vi "ScanAction.vi"(8 "error in (no error)":errorcluster caption="entrée d'erreur (pas d'erreur)", 9 "IndicePoint":i32, 10 "Dir":bool, 11 "Tools In":refnum<class "CoboltMLD.lvclass"> caption="DNL_LabVIEW Object in") -> (0 "error out":errorcluster caption="sortie d'erreur", 2 "ScanParsOut":dbl[](array[numeric]), 3 "Tools Out":refnum<class "CoboltMLD.lvclass"> caption="DNL_LabVIEW Object out")   [LabVIEW 2019, in "CoboltMLD.lvclass"]
uses:
  CoboltMLD.lvclass
  C:/Programmes Labview/LabscanV1A/DevicesClass/BaseDevice/BaseDevice.lvclass
  CoboltMLD.lvclass/CoboltMLD.ctl
  <userlib>/GenProg/ReadValByRefU32.vi
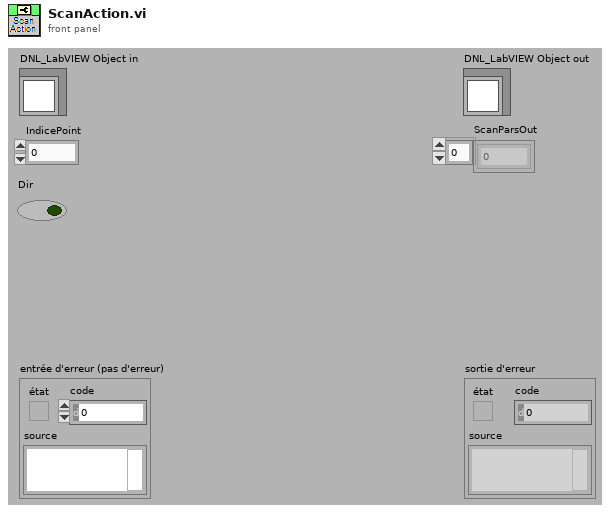
[diagram p1: front panel]
types:
  T1 = typedef "CoboltMLD.lvclass/CoboltMLD_Func.ctl" = enum16{"Power (mW)", "Freq (kHz)"}
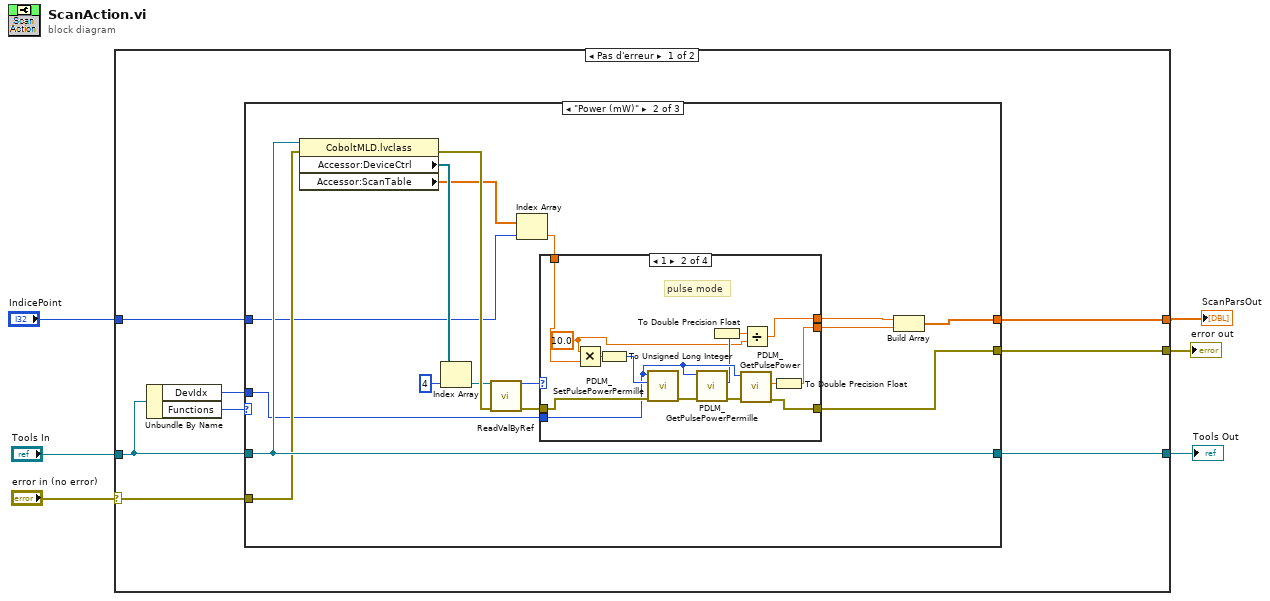
[diagram p0: block diagram]
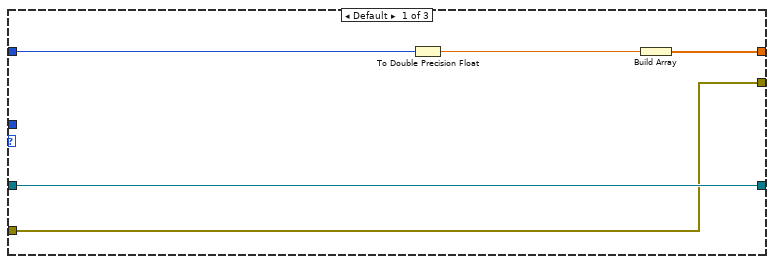
[diagram p2: hidden frame]
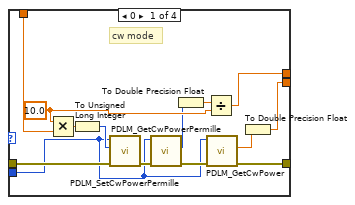
[diagram p3: hidden frame]
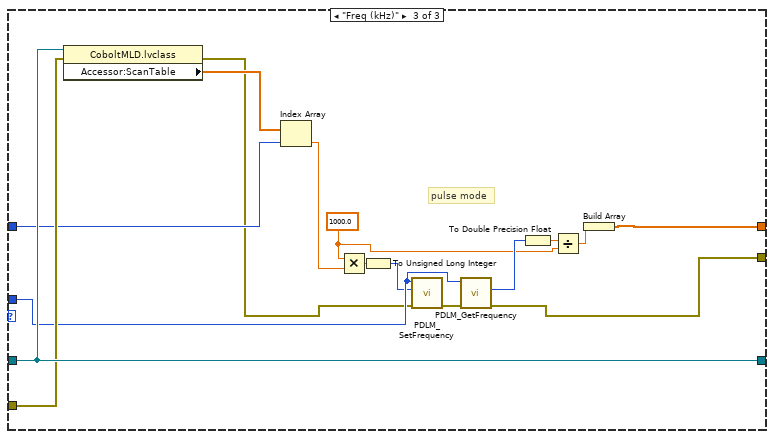
[diagram p6: hidden frame]
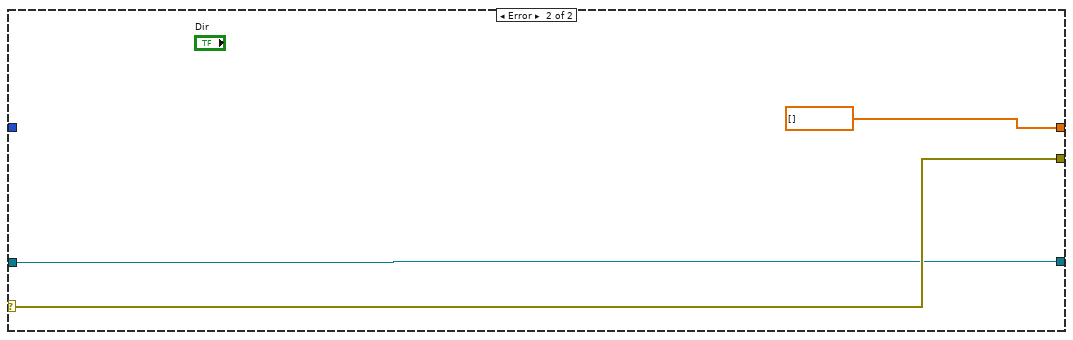
[diagram p7: hidden frame]
diagram:
  n1 = case shown="Pas d'erreur" "error in (no error)" {
    selector: "error in (no error)" -> [w11 w84]
    tunnel: "Tools In" -> [w12 w83]
    tunnel: [w10 dbl[] []] -> w1
    tunnel: [w9 w84] -> w4
    tunnel: [w8 w83] -> w3
    tunnel: "IndicePoint" -> [w13 _]
    frame No Error {
      n2 = Unbundle By Name(w12) -> ("DevIdx"=w7:i32, "Functions"=w14:T1)
      n3 = case shown="\"Power (mW)\"" w14 {
        tunnel: [w15 w35 w74] -> w10
        tunnel: w13 -> [w19 w26 w78]
        tunnel: [w17 w34 w81] -> w8
        tunnel: w12 -> [w17 w34 w81]
        tunnel: w11 -> [w16 w33 w80]
        tunnel: [w16 w22 w75] -> w9
        tunnel: w7 -> [_ w24 w76]
        frame Default {
          n4 = To Double Precision Float(number=w19) -> (double precision float=w18:dbl)
          n5 = Build Array(w18) -> (w15:dbl[])
        }
        frame "Power (mW)" {
          n6 = property class="CoboltMLD.lvclass"(reference=w34, error in=w33) -> (error out=w32:errorcluster, "Accessor:DeviceCtrl"=w31:refnum<vi>[], "Accessor:ScanTable"=w27:dbl[])  [unwired: 1 out]
          n7 = Index Array(array=w31, index=4 ("indice")) -> (element=w29:refnum<vi>)
          n8 = call-poly <userlib>:"ReadValByRef.vi"("Control Ref"=w29, "error in"=w32) -> ("Valeur"=w28:u32, "error out"=w23:errorcluster)  [unwired: 12 in]
          n9 = Index Array(array=w27, index=w26) -> (element=w25:dbl)
          n10 = case shown="1" w28 {
            tunnel: w25 -> [w47 w61 _ _]
            tunnel: w24 -> [w36 w54 _ _]
            tunnel: w23 -> [w49 w63 w64 w65]
            tunnel: [w43 w57 w64 w65] -> w22
            tunnel: [w37 w55 _ _] -> w21
            tunnel: [w39 w50 _ _] -> w20
            frame 0 {
              w42 = 10.0 ("x")
              # "cw mode"
              n11 = Multiply(x=w42, y=w47) -> (x*y=w48:dbl)
              n12 = To Unsigned Long Integer(number=w48) -> (unsigned 32bit integer=w46:u32)
              n13 = call <userlib>:"PDLM_SetCwPowerPermille.vi"("error in (no error)"=w49, "permille"=w46, "USBIdx"=w36) -> ("error out"=w45:errorcluster)  [unwired: 7 in, 1 out]
              n14 = call <userlib>:"PDLM_GetCwPowerPermille.vi"("error in (no error)"=w45, "USBIdx"=w36) -> ("error out"=w44:errorcluster, "permille"=w41:u32)  [unwired: 7 in, 1 out]
              n15 = To Double Precision Float(number=w41) -> (double precision float=w40:dbl)
              n16 = Divide(x=w40, y=w42) -> (x/y=w39:dbl)
              n17 = call <userlib>:"PDLM_GetCwPower.vi"("error in (no error)"=w44, "USBIdx"=w36) -> ("error out"=w43:errorcluster, "Power"=w38:sgl)  [unwired: 7 in, 1 out]
              n18 = To Double Precision Float(number=w38) -> (double precision float=w37:dbl)
            }
            frame 1 {
              w51 = 10.0 ("x")
              # "pulse mode"
              n19 = Multiply(x=w51, y=w61) -> (x*y=w62:dbl)
              n20 = To Unsigned Long Integer(number=w62) -> (unsigned 32bit integer=w60:u32)
              n21 = call <userlib>:"PDLM_SetPulsePowerPermille.vi"("error in (no error)"=w63, "permille"=w60, "USBIdx"=w54) -> ("error out"=w59:errorcluster)  [unwired: 7 in, 1 out]
              n22 = call <userlib>:"PDLM_GetPulsePowerPermille.vi"("error in (no error)"=w59, "USBIdx"=w54) -> ("error out"=w58:errorcluster, "permille"=w52:u32)  [unwired: 7 in, 1 out]
              n23 = To Double Precision Float(number=w52) -> (double precision float=w53:dbl)
              n24 = call <userlib>:"PDLM_GetPulsePower.vi"("error in (no error)"=w58, "USBIdx"=w54) -> ("error out"=w57:errorcluster, "Power"=w56:sgl)  [unwired: 7 in, 1 out]
              n25 = Divide(x=w53, y=w51) -> (x/y=w50:dbl)
              n26 = To Double Precision Float(number=w56) -> (double precision float=w55:dbl)
            }
            frame 2 {
            }
            frame Default {
            }
          }
          n27 = Build Array(w20, w21) -> (w35:dbl[])
        }
        frame "Freq (kHz)" {
          w67 = 1000.0 ("x")
          # "pulse mode"
          n28 = property class="CoboltMLD.lvclass"(reference=w81, error in=w80) -> (error out=w73:errorcluster, "Accessor:ScanTable"=w79:dbl[])  [unwired: 1 out]
          n29 = Index Array(array=w79, index=w78) -> (element=w77:dbl)
          n30 = Multiply(x=w67, y=w77) -> (x*y=w72:dbl)
          n31 = To Unsigned Long Integer(number=w72) -> (unsigned 32bit integer=w71:u32)
          n32 = call <userlib>:"PDLM_SetFrequency.vi"("error in (no error)"=w73, "freq"=w71, "USBIdx"=w76) -> ("error out"=w70:errorcluster)  [unwired: 7 in, 1 out]
          n33 = call <userlib>:"PDLM_GetFrequency.vi"("error in (no error)"=w70, "USBIdx"=w76) -> ("error out"=w75:errorcluster, "freq"=w68:u32)  [unwired: 7 in, 1 out]
          n34 = To Double Precision Float(number=w68) -> (double precision float=w69:dbl)
          n35 = Divide(x=w69, y=w67) -> (x/y=w66:dbl)
          n36 = Build Array(w66) -> (w74:dbl[])
        }
      }
    }
    frame Error {
    }
  }
  "error out" <- w4
  "Tools Out" <- w3
  "ScanParsOut" <- w1
